vi "Set Data Value.vi"(8 "error in (no error)":errorcluster, 9 "Flat Data":u8[](array[numeric]) format="%.0x", 11 "CIFTag in":refnum<class "CIF_CIPC_Chn_Double.lvclass">) -> (0 "error out":errorcluster, 1 "Updated":bool, 3 "CIFTag out":refnum<class "CIF_CIPC_Chn_Double.lvclass">)   [LabVIEW 2021, in "CIF_CIPC_Chn_Double.lvclass"]
uses:
  CIF_CIPC_Chn_Double.lvclass
  CIF_CIPC_Chn_Double.lvclass/CIF_CIPC_Chn_Double.ctl
  ChannelCommon/typedef/Errors.ctl
  <vilib>/CIF Foundation/CIF Utilities/Errors/Append Error Location.vi
  ChannelCommon/ChannelCommon.lvlib
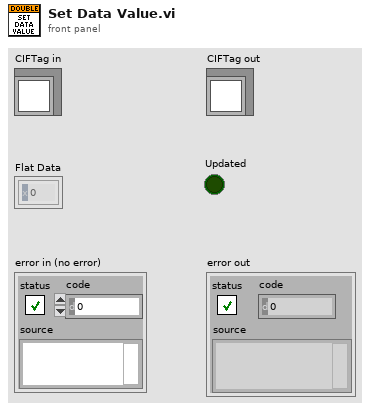
[diagram p1: front panel]
types:
  T1 = typedef "ChannelCommon.lvlib/Errors.ctl" = enum16{"gRPC Server Not Found", "Duplicate Channel", "Missing Channel", "Incorrect Type", "Flatten Error", "Unflatten Data", "Channel Length", "Plugin Connection", "gRPC Server Connection", "FIFO Unflatten", "Required Override", "Remove Not Found", "Not Supported"}
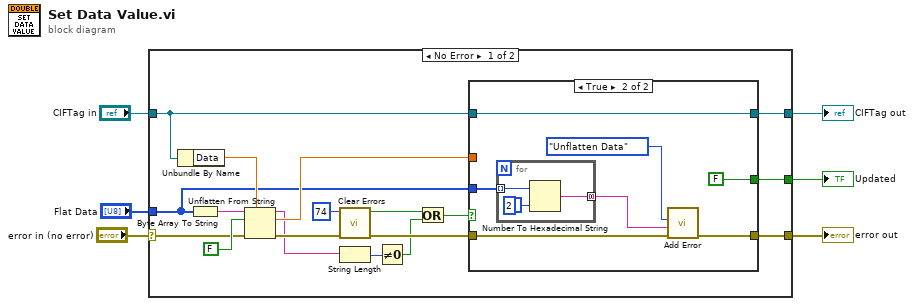
[diagram p0: block diagram]
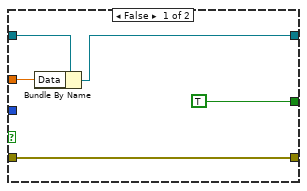
[diagram p2: hidden frame]
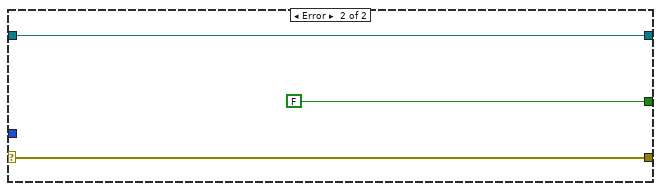
[diagram p3: hidden frame]
diagram:
  n1 = case shown="No Error" "error in (no error)" {
    selector: "error in (no error)" -> [w16 w42]
    tunnel: "Flat Data" -> [w13 _]
    tunnel: "CIFTag in" -> [w18 w41]
    tunnel: [w15 w42] -> w3
    tunnel: [w14 w41] -> w2
    tunnel: [w12 FALSE] -> w1
    frame No Error {
      n2 = Unbundle By Name(w18) -> ("Data"=w22:dbl)
      n3 = Byte Array To String(unsigned byte array=w13) -> (string=w24:string)
      n4 = Unflatten From String(type=w22, binary string=w24, data includes array or string size? (T)=FALSE, error in (no error)=w16) -> (rest of the binary string=w11:string, value=w17:dbl, error out=w21:errorcluster)  [unwired: 1 in]
      n5 = call <vilib>:"Clear Errors.vi"("error in (no error)"=w21, "specific error code to clear (0: all)"=74) -> ("error out"=w19:errorcluster, "specific error cleared?"=w9:bool)  [unwired: 4 in]
      n6 = String Length(string=w11) -> (length=w10:i32)
      n7 = Not Equal To 0?(x=w10) -> (x != 0?=w8:bool)
      n8 = Or(x=w9, y=w8) -> (x .or. y?=w7:bool)
      n9 = case shown="True" w7 {
        tunnel: w19 -> [w27 w36]
        tunnel: w18 -> [w29 w33]
        tunnel: w17 -> [w28 _]
        tunnel: [w27 w35] -> w15
        tunnel: [w26 w33] -> w14
        tunnel: w13 -> [_ w32]
        tunnel: [TRUE FALSE] -> w12
        frame False {
          n10 = Bundle By Name(cluster=w29, "Data"=w28) -> (w26:refnum<class "CIF_CIPC_Chn_Double.lvclass">)
        }
        frame True {
          n11 = for {
            tunnel: w32 -> [w39] mode=indexing
            tunnel: [w38] -> w31 mode=concatenating
            n12 = Number To Hexadecimal String(1:i16 2 ("width (-)"), 2:w39) -> (0:w38:string)
          }
          n13 = call "Add Error.vi"("error in (no error)"=w36, "String to Append"=w31, "Error"=Errors."Unflatten Data") -> ("error out"=w35:errorcluster)  [unwired: 8 in]
        }
      }
    }
    frame Error {
    }
  }
  "CIFTag out" <- w2
  "Updated" <- w1
  "error out" <- w3
